vi "Serialize.vi"(8 "error in (no error)":errorcluster, 10 "Item Info":refnum<class "XML Node.lvclass">, 11 "Build Package Item in":refnum<class "VIPM Item.lvclass">) -> (0 "error out":errorcluster, 2 "Serialization Version":string)   [LabVIEW 2019, in "VIPM.lvlib" / "VIPM Item.lvclass"]
uses:
  VIPM Item.lvclass
  libs/Solution.lvlibp/Solution/XML Reader/XML Node.lvclass
  VIPM Item.lvclass/VIPM Item.ctl
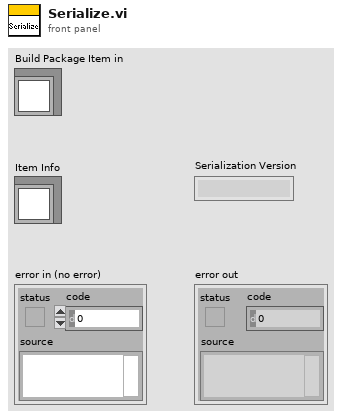
[diagram p1: front panel]
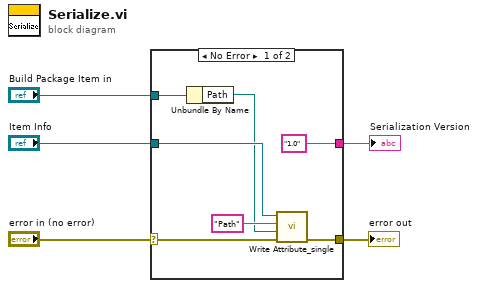
[diagram p0: block diagram]
diagram:
  n1 = case shown="No Error" "error in (no error)" {
    selector: "error in (no error)" -> [w11 w13]
    tunnel: "Item Info" -> [w12 _]
    tunnel: [w10 w13] -> w3
    tunnel: "Build Package Item in" -> [w8 _]
    tunnel: ["1.0" ("Serialization Version") _] -> w1
    frame No Error {
      n2 = Unbundle By Name(w8) -> ("Path"=w7:path)
      n3 = call "Write Attribute_single.vi"("error in (no error)"=w11, "Value"=w7, "Name"="Path", "XML Node in"=w12) -> ("error out"=w10:errorcluster)  [unwired: 7 in]
    }
    frame Error {
    }
  }
  "error out" <- w3
  "Serialization Version" <- w1
